vi "Blocker.vi"(7 "block?":bool, 8 "Error in":errorcluster) -> (0 "Error Out":errorcluster)   [LabVIEW 2018]
uses:
  type defines/Pause action.ctl
  Controls/FGV Actions.ctl
  Controls/Queue Manager Actions.ctl
  Controls/QueueNames.ctl
  Controls/MessagePacket.ctl
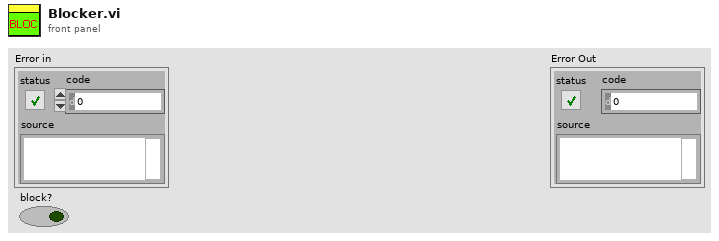
[diagram p1: front panel]
types:
  T1 = typedef "MessagePacket.ctl" = cluster{"Message":string, "Parameter":variant}
  T2 = typedef "QueueNames.ctl" = enum16{"Main GUI", "Main Scan Processor", "Main Processing", "Main Saving", "Main Display", "Main Table Stage GUI", "Main Table Stage Proc.", "Scan Engine", "Vibratome GUI", "Vibratome Processor", "Slice Engine"}
  T3 = typedef "Queue Manager Actions.ctl" = enum16{"Init", "Enqueue", "Enqueue All", "Preview Queue", "Dequeue", "Get Status", "Flush Queue", "Flush All Queues", "Release All Queues", "Release Queue", "Enqueue at Opposite End"}
  T4 = typedef "FGV Actions.ctl" = enum16{"Init", "Set", "Get", "Clear"}
  T5 = typedef "Pause action.ctl" = enum16{"Init", "get", "set"}
  T6 = typedef "System Parameters.ctl" = cluster{"Optical Parameters":T7, "Vibratome":T8, "Table Stages":T9, "Imaging Parameter":T12, "Galvo HW Parameters":cluster{"Analog Out Channel":tag, "Min Voltage":dbl, "Max Voltage":dbl, "Pixel Clock Source":tag, "Sample Rate":dbl, "Line Clock Out Ch":tag, "2P ready check":tag}, "Alazar parameters":T14, "Mosaic Paramter":T21, "Manual Controls":T22, "Z stage setting":T26, "Attenuator":T27, "Pause?":bool}
  T7 = typedef "Optical Parameters.ctl" = cluster{"Obj. Focal Length [mm]":dbl, "Scan Lens EFL[mm]":dbl, "Tube Lens EFL[mm]":dbl, "Galvo V Range (+/-)":dbl, "Galvo Max Half Angle [Deg]":dbl, "Max Galvo Range[%]":dbl}
  T8 = typedef "Vibratome Parameters.ctl" = cluster{"Pre Cut Dwell [s]":dbl, "Blade Frequency [RPM]":u16, "Slice Speed [mm/s]":dbl, "Post Cut Dwell [s]":dbl, "Ramp Time [s]":dbl, "Start X [mm]":dbl, "Start Y [mm]":dbl, "Slice Length [mm]":dbl, "Slice Axis":enum16{"X Axis", "Y Axis", "Z Axis"}, "Controller VISA Ref":refnum<visa-resource-name>}
  T9 = typedef "Translation Stage Parameters.ctl" = cluster{"X Stage":T10, "Y Stage":T10, "Z Stage":T10, "Attenuator":T10}
  T10 = typedef "Translation Stage Cluster.ctl" = cluster{"Position":dbl, "Is.Enabled?":bool, "Is.Connected?":bool, "Device SN":string, "AccelerationMaximum":dbl, "VelocityMaximum":dbl, "Acceleration":dbl, "Velocity":dbl, "waitTimeout (ms)":i32, "Model":T11, "Is.Homed?":bool, "MOVE":bool}
  T11 = typedef "Translation Stage Types.ctl" = enum16{"None", "Thorlabs LTS", "Thorlabs MLJ"}
  T12 = typedef "Imaging Parameters.ctl" = cluster{"Raster Scan Direction":T13, "Pixel Dwell Time [Clock Cycles]":u16, "Flyback Time [Clock Cycles]":u16, "XY Center [um]":cluster{"X":dbl, "Y":dbl}, "Pixel Step Size [um] X":dbl, "XY Image Size":enum16{"32 x 32", "64 x 64", "128 x 128", "256 x 256", "512 x 512", "1024 x 1024", "2048 x 2048"}, "Custom":bool, "Custom Size":cluster{"X":u16, "Y":u16}, "Line Averages":u16, "Pixel Step Size [um] Y":dbl}
  T13 = typedef "Scan Direction.ctl" = enum16{"Uni Directional", "Bi Directional", "None"}
  T14 = typedef "Alazar parameters.ctl" = cluster{"Trigger Settings":cluster{"General Trigger Settings":T15, "Trigger Engine 1":T16, "Trigger Engine 2":T16}, "Device ID":T17, "Ch A Input Control":T18, "Ch B Input Control":T18, "Acq Settings":T19, "Capture Clock":T20}
  T15 = typedef "General Trigger Settings.ctl" = cluster{"Trigger Operation":u32, "Coupling ID":u32, "Range ID":u32, "Delay":u32, "Timeout Ticks":u32, "Mode":u32, "Parameter":u32}
  T16 = typedef "Trigger Engine Controls.ctl" = cluster{"Trigger Engine":u32, "Source":u32, "Slope":u32, "Level":u32}
  T17 = typedef "Alazar Device ID.ctl" = cluster{"System ID":u32, "Board ID":u32}
  T18 = typedef "Channel Input Controls.ctl" = cluster{"Channel":u8, "Coupling":u32, "Range":u32, "Impedance":u32}
  T19 = typedef "Alazar Acquisition Settings.ctl" = cluster{"Record Length":u32, "Offset":u32, "Records Per Buffer":u32, "Records Count (Records/Acq)":u32, "Window Type":u32, "Footer":u32, "Samples per record":u32, "Output Format":u32}
  T20 = typedef "Clock Controls.ctl" = cluster{"Sample Rate":u32, "Decimation":u32, "Source":u32, "Edge":u32}
  T21 = typedef "Mosaic Parameter.ctl" = cluster{"X Axis":cluster{"Start [mm]":dbl, "Steps [pts]":dbl, "End [mm]":dbl}, "Y Axis":cluster{"Start [mm]":dbl, "Steps [pts]":dbl, "End [mm]":dbl}, "Scan Pattern":enum16{"Uni-directional", "Bi-Directional", "Spiral Out", "Spiral In"}, "Overlap Options":cluster{"Overlap Type":enum16{"No Overlap", "X Only", "Y Only", "X and Y"}, "Percent Overlap":u8, "Justify":enum16{"Start", "Center", "End"}}}
  T22 = typedef "Manual Controls.ctl" = cluster{"Data Path":path, "Save parameters":T23, "Acquisition mode":T24, "PSOCT Channel":u32, "Save data?":bool, "AIP rotation angle":dbl, "Outgoing Mail Server (SMTP)":string, "Email":string, "Password":string, "Carrier 1":enum16{"T-Mobile", "AT&T", "Verizon", "Sprint"}, "phone number 1":string, "Subject":string, "Message":string, "Carrier 2":enum16{"T-Mobile", "AT&T", "Verizon", "Sprint"}, "phone number 2":string, "Outputs for GPU FFT":T25, "First Slice #":i32}
  T23 = typedef "FFT parameters.ctl" = cluster{"start pixel":i32, "#pixels to save":i32}
  T24 = typedef "FFT mode.ctl" = enum16{"ThorOCT B line", "ThorOCT Spectral", "ThorOCT FFT", "Alazar B line", "Alazar FFT", "GPU FFT", "Alazar Spectral", "Simulation", "auto adjust focus", "Save all"}
  T25 = typedef "GPU FFT outputs.ctl" = enum16{"Amp + Phase diff", "Amp + Phase", "Amp only"}
  T26 = typedef "Vibratome Param.ctl" = cluster{"first cut height(mm)":dbl, "cut thickness[um]":u32[], "#cycles":u16, "PSOCT thickness(um)":u32[], "First image height(mm)":dbl, "Pause?":bool[], "Z0":dbl, "fixed Z0?":bool, "Cut_aft_2P?(leave empty if no 2P)":bool[], "2P thickness(um) (leave empty if not used)":u32[], "2P_cover_all_depth? (leave empty if no 2P)":bool[]}
  T27 = typedef "attenuator.ctl" = cluster{"Power after Objective (recalibrate every 6 month)":dbl[]}
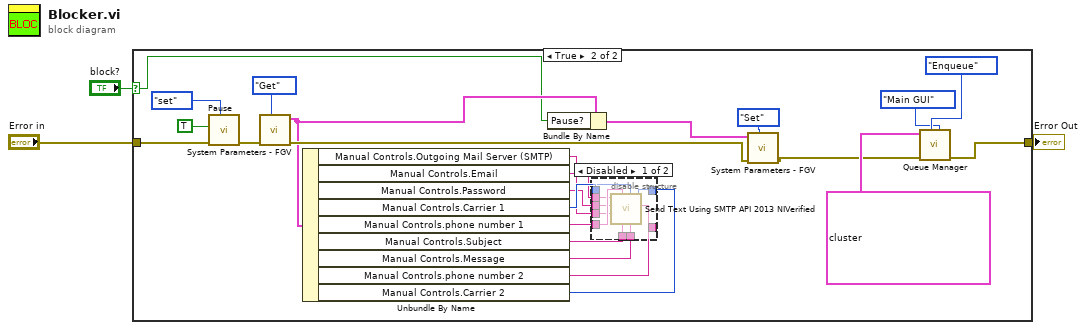
[diagram p0: block diagram]
diagram:
  n1 = case shown="True" "block?" {
    selector: "block?" -> [_ w11]
    tunnel: "Error in" -> [w4 w26]
    tunnel: [w4 w5] -> w2
    frame False {
    }
    frame True {
      n2 = call "Pause.vi"("action"=Pause_action."set", "error in"=w26, "Pause!"=TRUE) -> ("error out"=w25:errorcluster)  [unwired: 7 in, 1 out]
      n3 = call "System Parameters - FGV.vi"("Actions"=FGV_Actions."Get", "Error In"=w25) -> ("Error Out"=w13:errorcluster, "System Parameters [Out]"=w12:T6)  [unwired: 8 in]
      n4 = Unbundle By Name(w12) -> ("Manual Controls.Outgoing Mail Server (SMTP)"=w17:string, "Manual Controls.Email"=w21:string, "Manual Controls.Password"=w20:string, "Manual Controls.Carrier 1"=w23:enum16{"T-Mobile", "AT&T", "Verizon", "Sprint"}, "Manual Controls.phone number 1"=w22:string, "Manual Controls.Subject"=w19:string, "Manual Controls.Message"=w18:string, "Manual Controls.phone number 2"=w16:string, "Manual Controls.Carrier 2"=w15:enum16{"T-Mobile", "AT&T", "Verizon", "Sprint"})
      n5 = Bundle By Name(cluster=w12, "Pause?"=w11) -> (w10:T6)
      n6 = disable-structure shown="Disabled" {
        disable-tunnel: w23 -> [w37 _]
        disable-tunnel: w22 -> [w36 _]
        disable-tunnel: w21 -> [w35 _]
        disable-tunnel: w20 -> [w34 _]
        disable-tunnel: w19 -> [w33 _]
        disable-tunnel: w18 -> [w32 _]
        disable-tunnel: w17 -> [w31 _]
        disable-tunnel: w16 -> [w30 _]
        disable-tunnel: w15 -> [w29 _]
        frame Disabled {
          n7 = call "Send Text Using SMTP API 2013 NIVerified.vi"("phone number 2"=w30, "Carrier 2"=w29, "Body"=w32, "Carrier 1"=w37, "Subject"=w33, "phone number 1"=w36, "Outgoing Mail Server (SMTP)"=w31, "Password"=w34, "Email"=w35) -> ()  [unwired: 3 in]
        }
        frame Enabled {
        }
      }
      n8 = call "System Parameters - FGV.vi"("Actions"=FGV_Actions."Set", "Error In"=w13, "System Parameters [In]"=w10) -> ("Error Out"=w6:errorcluster)  [unwired: 7 in, 1 out]
      n9 = call "Queue Manager.vi"("Queue Name"=QueueNames."Main GUI", "Action"=Queue_Manager_Actions."Enqueue", "Error In"=w6, "Message Packet Array"=T1[] [{"Message"="Update User Settings", "Parameter"=variant}, {"Message"="Wait for User Input", "Parameter"=variant}]) -> ("Error Out"=w5:errorcluster)  [unwired: 3 in, 4 out]
    }
  }
  "Error Out" <- w2
